vi "getTemp.vi"(8 "error_in":errorcluster, 11 "VISA_in":refnum<visa-resource-name>) -> (0 "error_out":errorcluster, 2 "temp_out":dbl, 3 "VISA_out":refnum<visa-resource-name>)   [LabVIEW 2017]
uses:
  <vilib>/Instr/_visa.llb/VISA Configure Serial Port (Instr).vi
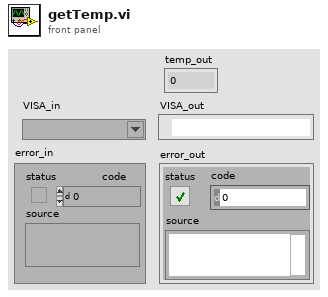
[diagram p1: front panel]
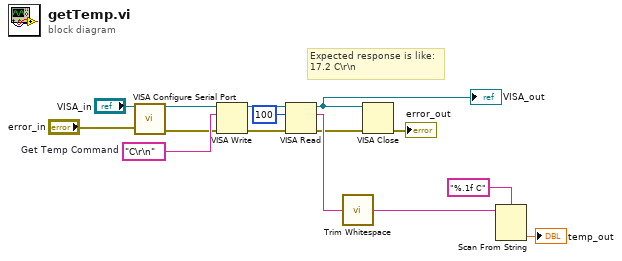
[diagram p0: block diagram]
diagram:
  w15 = "C\r\n"  # Get Temp Command
  # "Expected response is like:\n17.2 C\\r\\n"
  n1 = call-poly "VISA Configure Serial Port"("VISA resource name"="VISA_in", "error in (no error)"="error_in") -> ("VISA resource name out"=w9:refnum<visa-resource-name>, "error out"=w8:errorcluster)  [unwired: 12 in]
  n2 = VISA Write(VISA resource name=w9, write buffer=w15, error in (no error)=w8) -> (VISA resource name out=w7:refnum<visa-resource-name>, error out=w5:errorcluster)  [unwired: 1 out]
  n3 = VISA Read(VISA resource name=w7, byte count=u32 100, error in (no error)=w5) -> (VISA resource name out=w6:refnum<visa-resource-name>, read buffer=w14:string, error out=w4:errorcluster)  [unwired: 1 out]
  "VISA_out" <- w6
  n4 = call <vilib>:"Trim Whitespace.vi"("string"=w14) -> ("trimmed string"=w13:string)  [unwired: 1 in]
  n5 = VISA Close(VISA resource name=w6, error in (no error)=w4) -> (error out=→"error_out":errorcluster)
  n6 = Scan From String(format string="%.1f C", input string=w13) -> (output 1=→"temp_out":dbl)  [unwired: 3 in, 3 out]
